vi "Programming Assignment.vi"() -> ()   [LabVIEW 2020]
panel:
  out "?":dbl[](array[numeric])
  in  "Auto-pick":bool
  in  "Done":bool
  in  "Play":bool
  out "Bank":dbl
  out "Winnings":dbl
  in  "Bet":dbl min=0.0 max=50.0 step=1.0
  out "Results":dbl[](array[numeric])
  in  "Picks (0-99)":dbl[](array[numeric]) min=0.0 max=99.0 step=1.0
  # "Welcome"
  # "BET MORE WIN MORE"
  # "Wins = bet * number matched * 2 ^number matched"
  # "Play"
  # "Auto Pick"
  # "Done"
  # "Auto Pick"
  # "More numbers match \nMore money you win"
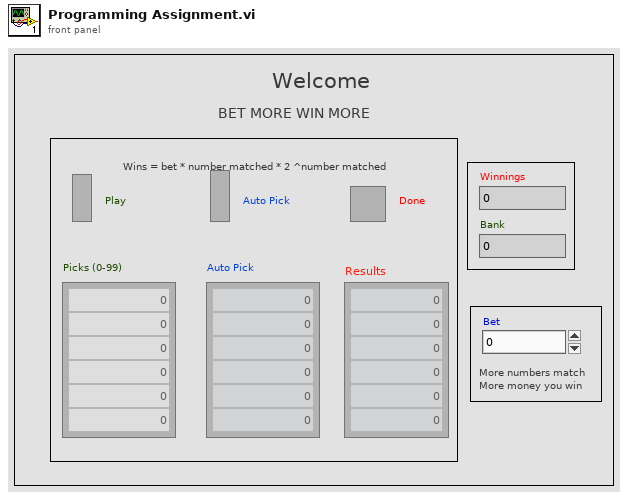
[diagram p1: front panel]
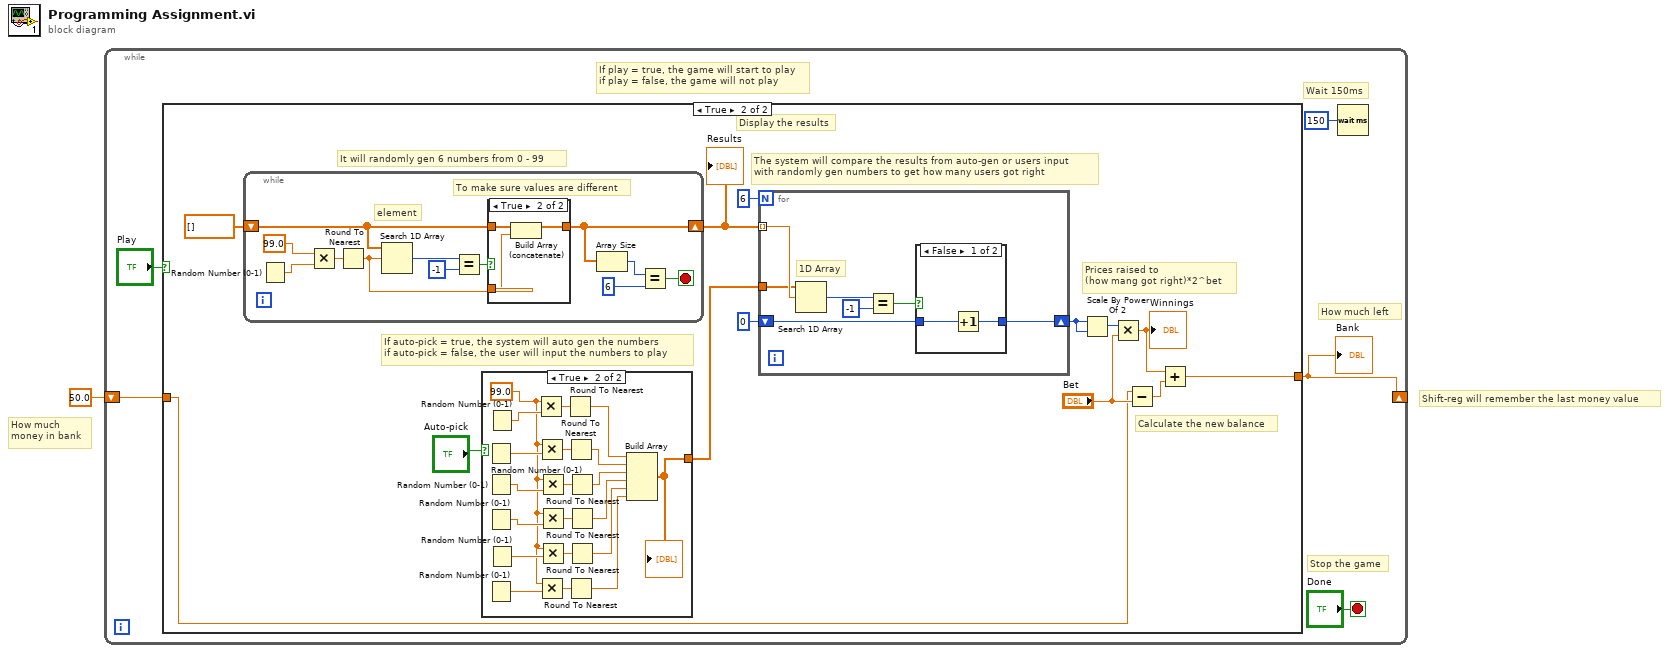
[diagram p0: block diagram]
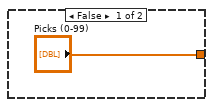
[diagram p3: hidden frame]
diagram:
  # "Shift-reg will remember the last money value"
  # "How much\nmoney in bank"
  n1 = while {
    shift-right: [w4] -> _
    shift-left: 50.0 -> [w5]
    stop <- "Done" stop-if-true
    # "How much left"
    # "Stop the game"
    # "Wait 150ms"
    # "If play = true, the game will start to play\nif play = false, the game will not play"
    n2 = case shown="True" "Play" {
      tunnel: w5 -> [w7 w10]
      tunnel: [w7 w12] -> w4
      frame False {
      }
      frame True {
        # "Calculate the new balance"
        # "Prices raised to\n(how mang got right)*2^bet"
        # "The system will compare the results from auto-gen or users input\nwith randomly gen numbers to get how many users got right"
        # "If auto-pick = true, the system will auto gen the numbers\nif auto-pick = false, the user will input the numbers to play"
        # "Display the results"
        # "It will randomly gen 6 numbers from 0 - 99"
        n3 = while {
          shift-right: [w55] -> w18
          shift-left: dbl[] [] -> [w56]
          stop <- w52 stop-if-true
          # "To make sure values are different"
          # "element"
          n4 = Random Number (0-1)() -> (number: 0 to 1=w61:dbl)
          n5 = Multiply(x=99.0, y=w61) -> (x*y=w63:dbl)
          n6 = Round To Nearest(number=w63) -> (nearest integer value=w57:dbl)
          n7 = Search 1D Array(1D array=w56, element=w57) -> (index of element=w59:i32)  [unwired: 1 in]
          n8 = Equal?(x=w59, y=-1) -> (x = y?=w58:bool)
          n9 = case shown="True" w58 {
            tunnel: w57 -> [_ w67]
            tunnel: [w64 w66] -> w55
            tunnel: w56 -> [w64 w65]
            frame False {
            }
            frame True {
              n10 = Build Array (concatenate)(w65, w67) -> (w66:dbl[])
            }
          }
          n11 = Array Size(array=w55) -> (size(s)=w54:i32)
          n12 = Equal?(x=w54, y=6) -> (x = y?=w52:bool)
        }
        "Results" <- w18
        n13 = case shown="True" "Auto-pick" {
          tunnel: ["Picks (0-99)" w22] -> w8
          frame False {
          }
          frame True {
            w29 = 99.0
            n14 = Random Number (0-1)() -> (number: 0 to 1=w34:dbl)
            n15 = Random Number (0-1)() -> (number: 0 to 1=w33:dbl)
            n16 = Random Number (0-1)() -> (number: 0 to 1=w32:dbl)
            n17 = Random Number (0-1)() -> (number: 0 to 1=w30:dbl)
            n18 = Random Number (0-1)() -> (number: 0 to 1=w40:dbl)
            n19 = Random Number (0-1)() -> (number: 0 to 1=w31:dbl)
            n20 = Multiply(x=w29, y=w40) -> (x*y=w41:dbl)
            n21 = Multiply(x=w29, y=w34) -> (x*y=w39:dbl)
            n22 = Multiply(x=w29, y=w30) -> (x*y=w35:dbl)
            n23 = Multiply(x=w29, y=w33) -> (x*y=w38:dbl)
            n24 = Multiply(x=w29, y=w32) -> (x*y=w37:dbl)
            n25 = Multiply(x=w29, y=w31) -> (x*y=w36:dbl)
            n26 = Round To Nearest(number=w41) -> (nearest integer value=w28:dbl)
            n27 = Round To Nearest(number=w39) -> (nearest integer value=w27:dbl)
            n28 = Round To Nearest(number=w35) -> (nearest integer value=w23:dbl)
            n29 = Round To Nearest(number=w38) -> (nearest integer value=w26:dbl)
            n30 = Round To Nearest(number=w37) -> (nearest integer value=w25:dbl)
            n31 = Round To Nearest(number=w36) -> (nearest integer value=w24:dbl)
            n32 = Build Array(w28, w27, w26, w25, w24, w23) -> (w22:dbl[])
            "?" <- w22
          }
        }
        n33 = for {
          N: 6 -> [_]
          tunnel: w18 -> [w46] mode=indexing
          shift-right: [w44] -> w16
          shift-left: 0 -> [w43]
          tunnel: w8 -> [w42]
          # "1D Array"
          n34 = Search 1D Array(1D array=w42, element=w46) -> (index of element=w47:i32)  [unwired: 1 in]
          n35 = Equal?(x=w47, y=-1) -> (x = y?=w45:bool)
          n36 = case shown="False" w45 {
            tunnel: [w50 w51] -> w44
            tunnel: w43 -> [w49 w51]
            frame False {
              n37 = Increment(x=w49) -> (x+1=w50:i32)
            }
            frame True {
            }
          }
        }
        n38 = Scale By Power Of 2(n=w16, x=w16) -> (x*2^n=w15:i32)
        n39 = Multiply(x=w15, y="Bet") -> (x*y=w13:dbl)
        "Winnings" <- w13
        n40 = Subtract(x=w10, y="Bet") -> (x-y=w14:dbl)
        n41 = Add(x=w13, y=w14) -> (x+y=w12:dbl)
      }
    }
    "Bank" <- w4
    n42 = Wait (ms)(milliseconds to wait=u32 150) -> ()  [unwired: 1 out]
  }
